vi "Generate Sequence.vi"(8 "error in (no error)":errorcluster, 11 "Toggle 8 in":refnum<class "Toggle 8.lvclass">) -> (0 "error out":errorcluster, 3 "Toggle 8 out":refnum<class "Toggle 8.lvclass">)   [LabVIEW 2020, in "Toggle 8.lvclass"]
uses:
  Toggle 8.lvclass
  C:/Sandbox/Git_Sandbox/WiSpry Test Framework source code (LV20)/WiSpry Test Framework/Devices/Device.lvclass
  PIC-device/PIC-Device.lvclass
panel:
  in  "CP Voltage":i32[](array[ring])=[23] items=["CP 24V", "CP 26V", "CP 28V", "CP 30V", "CP 31V", "CP 32V", "CP 33V", "CP 34V", "CP 35V", "CP 36V", "CP 37V", "CP 38V", "CP 39V", "CP 40V", "CP 41V", "CP 42V", "CP 43V", "CP 44V", "CP 45V", "CP 46V", "CP 47V", "CP 48V", "CP 49V", "CP 50V", "CP 51V", "CP 52V", "CP 53V", "CP 54V", "CP 56V", "CP 58V", "CP 60V", "CP 62V"]
  out "Measure":string[](array[string])
  out "Initialize":string[](array[string])
  out "Boolean array":bool[][](array[boolean])
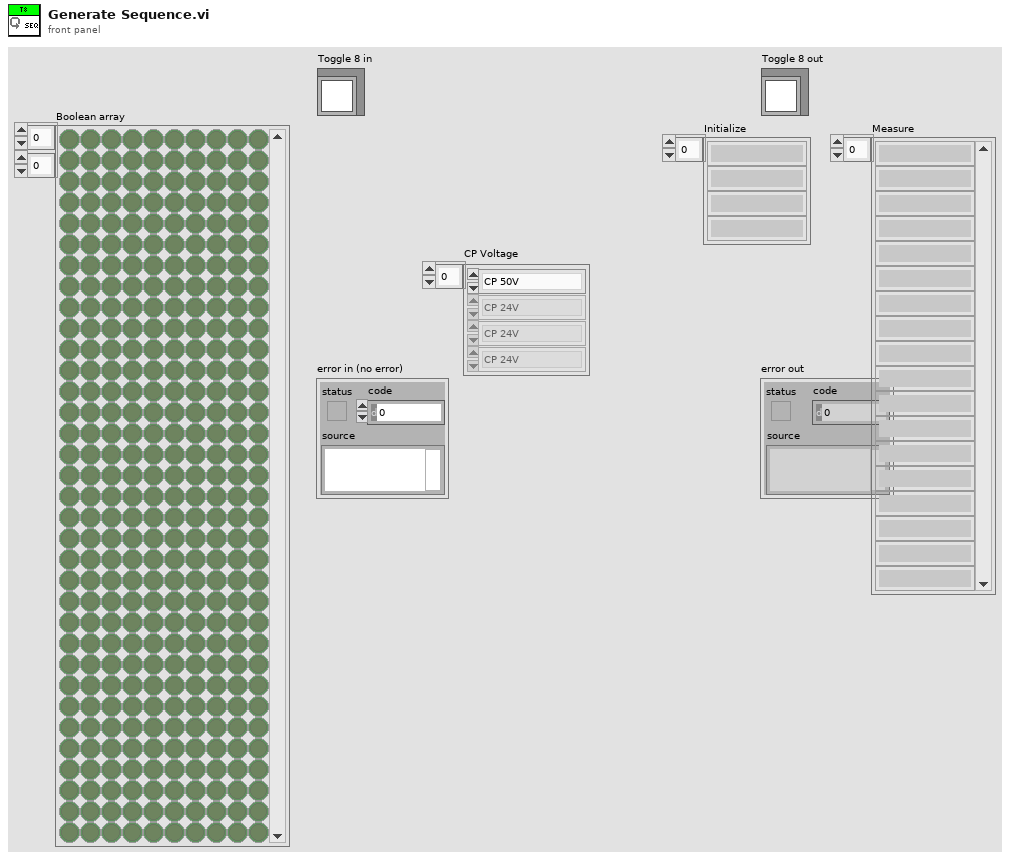
[diagram p1: front panel]
types:
  T1 = typedef "Toggle 8.lvclass/Test Sequence.ctl" = cluster{"CP values":string, "Charge Pump values":enum16{"CP 24V", "CP 26V", "CP 28V", "CP 30V", "CP 31V", "CP 32V", "CP 33V", "CP 34V", "CP 35V", "CP 36V", "CP 37V", "CP 38V", "CP 39V", "CP 40V", "CP 41V", "CP 42V", "CP 43V", "CP 44V", "CP 45V", "CP 46V", "CP 47V", "CP 48V", "CP 49V", "CP 50V", "CP 51V", "CP 52V", "CP 53V", "CP 54V", "CP 56V", "CP 58V", "CP 60V", "CP 62V"}[], "Charge Pump":T2[], "Control individual beams":bool, "OTP/beam values":dbl[], "Capa settings":T2[], "OTP Values string":string}
  T2 = typedef "PIC-Device.lvclass/Register to Write.ctl" = cluster{"Register":u32, "Value":u32, "Dev Address":u32, "Physical Adress":u32}
  T3 = enum16{"CP 24V", "CP 26V", "CP 28V", "CP 30V", "CP 31V", "CP 32V", "CP 33V", "CP 34V", "CP 35V", "CP 36V", "CP 37V", "CP 38V", "CP 39V", "CP 40V", "CP 41V", "CP 42V", "CP 43V", "CP 44V", "CP 45V", "CP 46V", "CP 47V", "CP 48V", "CP 49V", "CP 50V", "CP 51V", "CP 52V", "CP 53V", "CP 54V", "CP 56V", "CP 58V", "CP 60V", "CP 62V"}[]
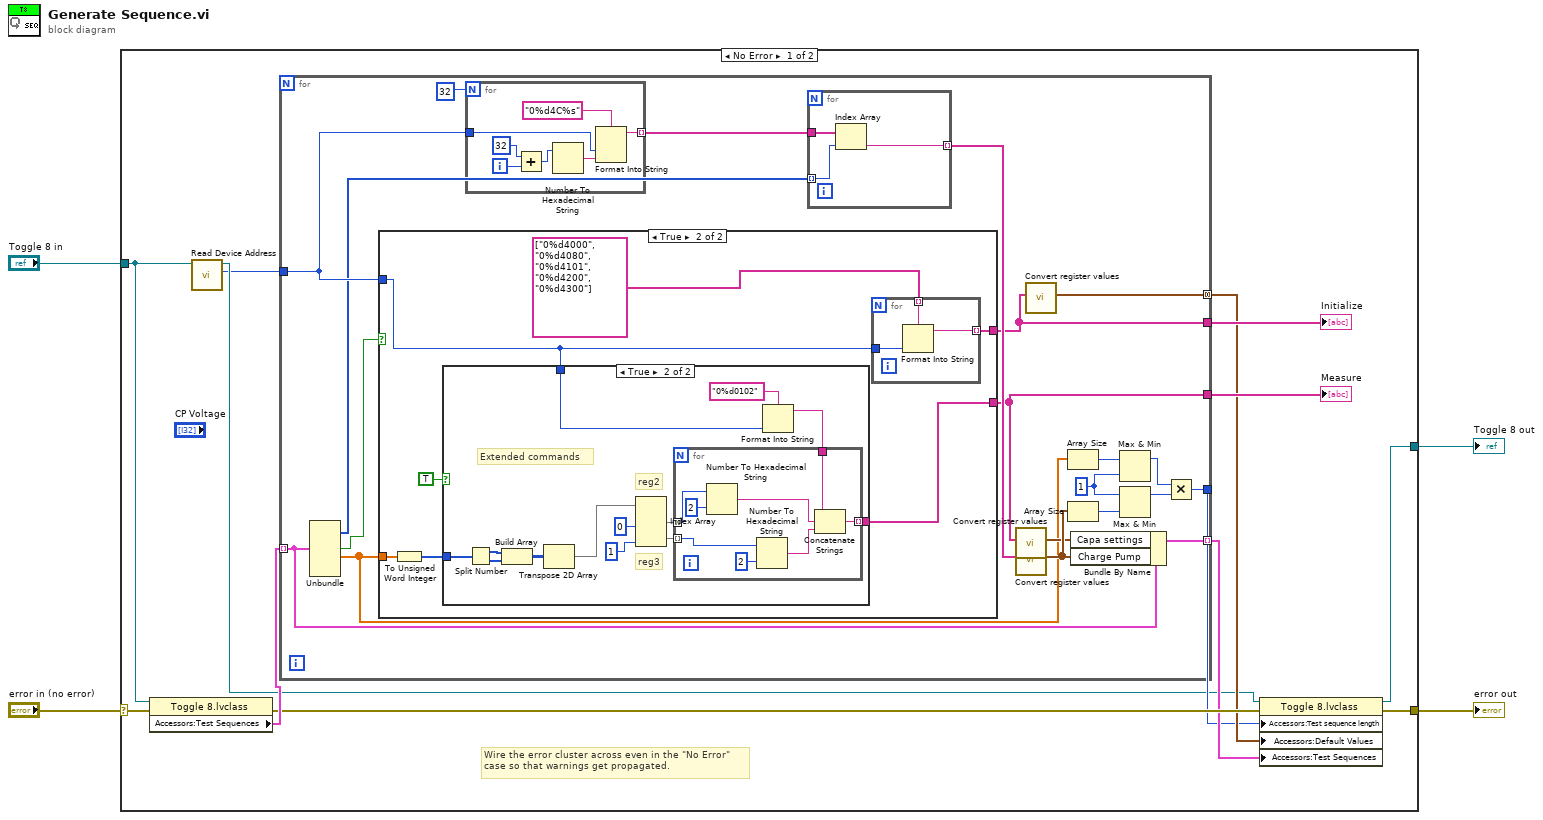
[diagram p0: block diagram]
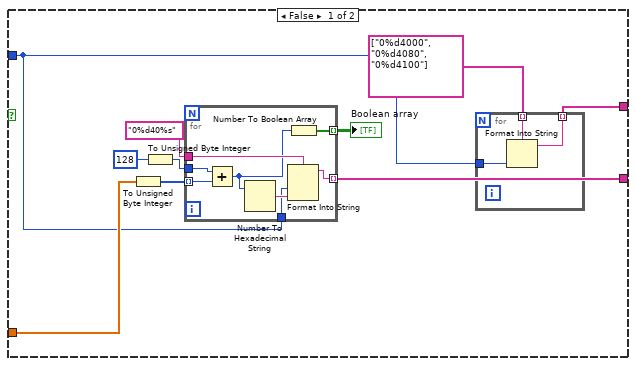
[diagram p2: hidden frame]
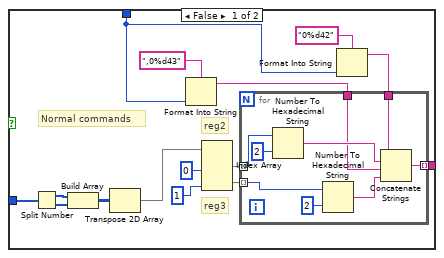
[diagram p3: hidden frame]
diagram:
  n1 = case shown="No Error" "error in (no error)" {
    selector: "error in (no error)" -> [w15 w125]
    tunnel: [w12 w125] -> w3
    tunnel: [w11 w124] -> w2
    tunnel: "Toggle 8 in" -> [w7 w124]
    frame No Error {
      # "Wire the error cluster across even in the \"No Error\"\ncase so that warnings get propagated."
      n2 = property class="Toggle 8.lvclass"(reference=w7, error in=w15) -> (error out=w13:errorcluster, "Accessors:Test Sequences"=w14:T1[])  [unwired: 1 out]
      n3 = call-dynamic "Read Device Address.vi"("PIC-Device in"=w7) -> ("Device Address"=w5:u8, "PIC-Device out"=w6:refnum<class "Toggle 8.lvclass">)  [unwired: 9 in]
      n4 = for {
        tunnel: [w33] -> w17
        tunnel: [w34] -> w16
        tunnel: w14 -> [w37] mode=indexing
        tunnel: [w36] -> w10 mode=indexing
        tunnel: [w32] -> w9 mode=concatenating
        tunnel: [w29] -> w8
        tunnel: w5 -> [w21]
        w24 = 1 ("x")
        n5 = Unbundle(w37) -> ("Charge Pump values"=w20:T3, "Control individual beams"=w18:bool, "OTP/beam values"=w19:dbl[])  [unwired: 4 out]
        n6 = case shown="True" w18 {
          tunnel: [w57 w75] -> w33
          tunnel: [w49 w71] -> w34
          tunnel: w19 -> [w55 w74]
          tunnel: w21 -> [w48 w70]
          frame False {
            n7 = To Unsigned Byte Integer(number=w55) -> (unsigned 8bit integer=w53:u8[])
            n8 = To Unsigned Byte Integer(number=u8 128) -> (unsigned 8bit integer=w51:u8)
            n9 = for {
              tunnel: w53 -> [w64] mode=indexing
              tunnel: "0%d40%s" -> [w68]
              tunnel: [w67] -> w56 mode=indexing
              tunnel: w51 -> [w66]
              tunnel: [w62] -> w57 mode=indexing
              tunnel: w48 -> [w61]
              n10 = Add(x=w66, y=w64) -> (x+y=w65:u8)
              n11 = Number To Hexadecimal String(2:w65) -> (0:w63:string)  [unwired: 1 in]
              n12 = Format Into String(format string=w68, w61, w63) -> (resulting string=w62:string)  [unwired: 2 in, 1 out]
              n13 = Number To Boolean Array(number=w65) -> (Boolean array=w67:bool[])
            }
            "Boolean array" <- w56
            n14 = for {
              tunnel: string[] ["0%d4000", "0%d4080", "0%d4100"] ("Opening sequence") -> [w60] mode=indexing
              tunnel: [w59] -> w49 mode=indexing
              tunnel: w48 -> [w58]
              n15 = Format Into String(format string=w60, w58) -> (resulting string=w59:string)  [unwired: 2 in, 1 out]
            }
          }
          frame True {
            n16 = To Unsigned Word Integer(number=w74) -> (unsigned 16bit integer=w73:u16[])
            n17 = case shown="True" TRUE {
              tunnel: [w90 w112] -> w75
              tunnel: w73 -> [w85 w107]
              tunnel: w70 -> [w76 w100]
              frame False {
                # "Normal commands"
                # "reg3"
                # "reg2"
                n18 = Split Number(x=w85) -> (hi(x)=w84:u8[], lo(x)=w83:u8[])
                n19 = Build Array(w84, w83) -> (w82:u8[][])
                n20 = Transpose 2D Array(2D array=w82) -> (transposed array=w81:u8[][])
                n21 = Format Into String(format string=",0%d43" ("string"), w76) -> (resulting string=w77:string)  [unwired: 2 in, 1 out]
                n22 = Index Array(array=w81, index (col) #1=0 ("disabled index (col)"), index (col) #2=1 ("disabled index (col)")) -> (element #1=w88:u8[], element #2=w89:u8[])  [unwired: 2 in]
                n23 = Format Into String(format string="0%d42" ("string"), w76) -> (resulting string=w79:string)  [unwired: 2 in, 1 out]
                n24 = for {
                  tunnel: w88 -> [w97] mode=indexing
                  tunnel: w89 -> [w93] mode=indexing
                  tunnel: [w99] -> w90 mode=indexing
                  tunnel: w79 -> [w92]
                  tunnel: w77 -> [w91]
                  n25 = Number To Hexadecimal String(1:i16 2 ("width (-)"), 2:w97) -> (0:w96:string)
                  n26 = Number To Hexadecimal String(1:i16 2 ("width (-)"), 2:w93) -> (0:w94:string)
                  n27 = Concatenate Strings(w92, w96, w91, w94) -> (w99:string)
                }
              }
              frame True {
                # "Extended commands"
                # "reg3"
                # "reg2"
                n28 = Split Number(x=w107) -> (hi(x)=w106:u8[], lo(x)=w105:u8[])
                n29 = Build Array(w106, w105) -> (w104:u8[][])
                n30 = Transpose 2D Array(2D array=w104) -> (transposed array=w103:u8[][])
                n31 = Index Array(array=w103, index (col) #1=0 ("disabled index (col)"), index (col) #2=1 ("disabled index (col)")) -> (element #1=w110:u8[], element #2=w111:u8[])  [unwired: 2 in]
                n32 = Format Into String(format string="0%d0102" ("string"), w100) -> (resulting string=w101:string)  [unwired: 2 in, 1 out]
                n33 = for {
                  tunnel: w110 -> [w118] mode=indexing
                  tunnel: w111 -> [w114] mode=indexing
                  tunnel: [w120] -> w112 mode=indexing
                  tunnel: w101 -> [w113]
                  n34 = Number To Hexadecimal String(1:i16 2 ("width (-)"), 2:w118) -> (0:w117:string)
                  n35 = Number To Hexadecimal String(1:i16 2 ("width (-)"), 2:w114) -> (0:w115:string)
                  n36 = Concatenate Strings(w113, w117, w115) -> (w120:string)
                }
              }
            }
            n37 = for {
              tunnel: string[] ["0%d4000", "0%d4080", "0%d4101", "0%d4200", "0%d4300"] ("Opening sequence") -> [w123] mode=indexing
              tunnel: [w122] -> w71 mode=indexing
              tunnel: w70 -> [w121]
              n38 = Format Into String(format string=w123, w121) -> (resulting string=w122:string)  [unwired: 2 in, 1 out]
            }
          }
        }
        n39 = for {
          N: 32 -> [_]
          tunnel: [w38] -> w22 mode=indexing
          tunnel: w21 -> [w40]
          i -> [w44]
          n40 = Add(x=32, y=w44) -> (x+y=w43:i32)
          n41 = Number To Hexadecimal String(2:w43) -> (0:w39:string)  [unwired: 1 in]
          n42 = Format Into String(format string="0%d4C%s", w40, w39) -> (resulting string=w38:string)  [unwired: 2 in, 1 out]
        }
        n43 = for {
          tunnel: w22 -> [w47]
          tunnel: w20 -> [w46] mode=indexing
          tunnel: [w45] -> w35 mode=indexing
          n44 = Index Array(array=w47, index=w46) -> (element=w45:string)
        }
        n45 = call "Convert register values.vi"("Register strings"=w33) -> ("Register clusters out"=w30:T2[])  [unwired: 9 in, 1 out]
        n46 = call "Convert register values.vi"("Register strings"=w35) -> ("Register clusters out"=w31:T2[])  [unwired: 9 in, 1 out]
        n47 = call "Convert register values.vi"("Register strings"=w34) -> ("Register clusters out"=w32:T2[])  [unwired: 9 in, 1 out]
        n48 = Array Size(array=w19) -> (size(s)=w26:i32)
        n49 = Array Size(array=w31) -> (size(s)=w27:i32)
        n50 = Bundle By Name(cluster=w37, "Capa settings"=w30, "Charge Pump"=w31) -> (w36:T1)
        n51 = Max & Min(x=w26, y=w24) -> (max(x,y)=w25:i32)  [unwired: 1 out]
        n52 = Max & Min(x=w24, y=w27) -> (max(x,y)=w28:i32)  [unwired: 1 out]
        n53 = Multiply(x=w25, y=w28) -> (x*y=w29:i32)
      }
      "Measure" <- w17
      "Initialize" <- w16
      n54 = property class="Toggle 8.lvclass"(reference=w6, error in=w13, "Accessors:Test sequence length"=w8, "Accessors:Default Values"=w9, "Accessors:Test Sequences"=w10) -> (reference out=w11:refnum<class "Toggle 8.lvclass">, error out=w12:errorcluster)
    }
    frame Error {
    }
  }
  "error out" <- w3
  "Toggle 8 out" <- w2
